vi "DisconnectAll.vi"(0 "reference in":refnum<class "SwitchBase.lvclass">, 5 "error in (no error)":errorcluster) -> (14 "reference in":refnum<class "SwitchBase.lvclass">, 19 "error out":errorcluster)   [LabVIEW 2022 SP3, in "SwitchBase.lvlib" / "SwitchBase.lvclass"]
uses:
  SwitchBase.lvclass
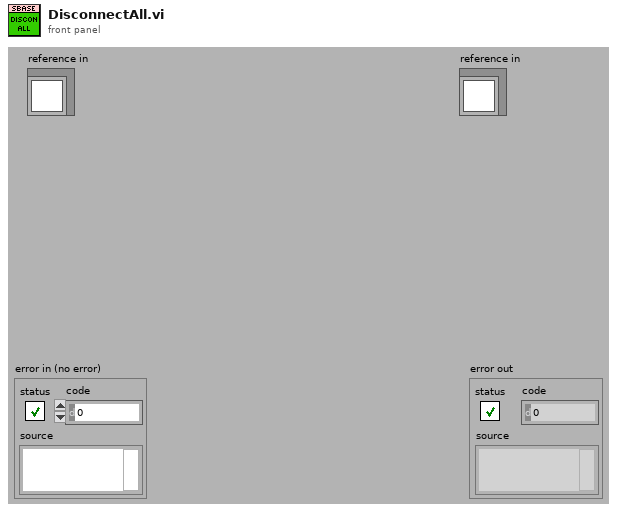
[diagram p1: front panel]
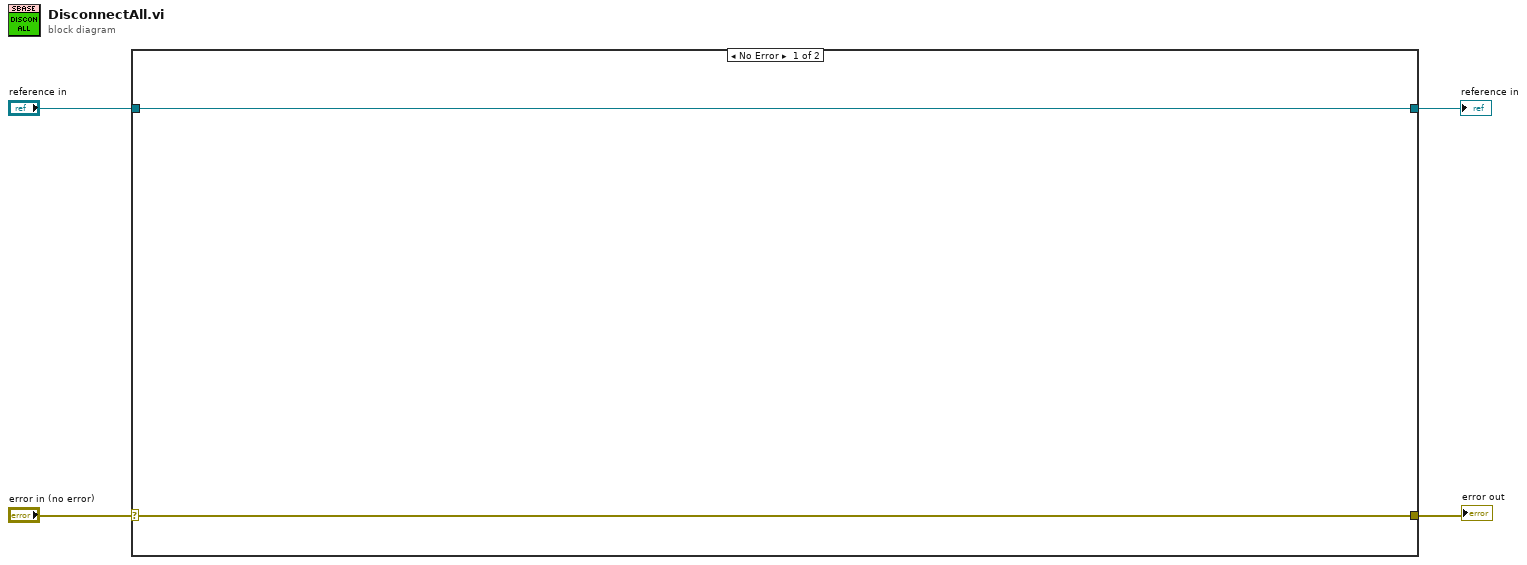
[diagram p0: block diagram]
diagram:
  n1 = case shown="No Error" "error in (no error)" {
    selector: "error in (no error)" -> [w6 w8]
    tunnel: [w6 w8] -> w3
    tunnel: [w5 w7] -> w1
    tunnel: "reference in" -> [w5 w7]
    frame No Error {
    }
    frame Error {
    }
  }
  "error out" <- w3
  "reference in" <- w1
